vi "Untitled 2.vi"() -> ()   [LabVIEW 2012, in "filenames.lvlib"]
uses:
  filenames.lvlib
panel:
  in  "stop":bool
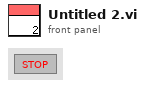
[diagram p1: front panel]
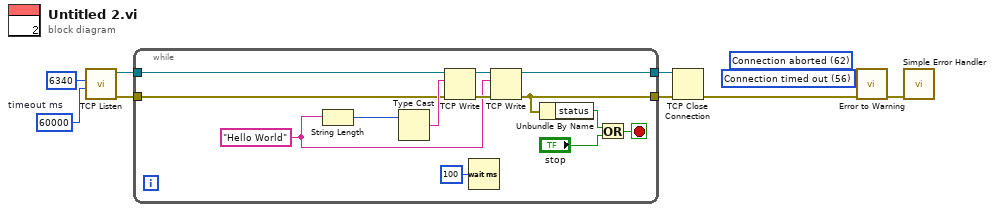
[diagram p0: block diagram]
diagram:
  w2 = 60000  # timeout ms
  w7 = 56 items=["No Error", "Argument Error", "Memory Full", "Out of Zone", "End of File", "File Already Open", "Generic File IO Error", "File Not Found", "File Permission Error", "Disk Full", "Duplicate Path", "Too Many Files Open", "Not Enabled", "Resource File Not Found", "Cannot Add Resource", "Resource Not Found", "Image Not Found", "Image Memory Error", "Pen Does Not Exist", "Config Bad Type", "Config Token Not Found", "Config Parse Error", "Config Memory Error", "Bad External Code Format", "Bad External Code Offset", "External Code Not Present", "Null Window", "Destroy Window Mixup", "Null Menu", "Print Aborted", "Bad Print Record", "Print Driver Error", "Windows Error During Print", "Memory Error During Print", "Print Dialog Error", "Generic Print Error", "Invalid Device Refnum", "Device Not Found", "Device Parameter Error", "Device Unit Error", "Can't Open Device", "Device Call Aborted", "Generic Error", "Cancelled By User", "Object ID Too Low", "Object ID Too High", "Object Not In Heap", "Unknown Heap", "Bad DefProc ID", "DefProc Not In Table", "Message Out Of Range", "Null Method", "Unknown Message", "Manager Call Not Supported", "Bad address", "Connection In progress", "Connection timed out", "Connection is already in progress", "Network attribute not supported", "Network error", "Address in use", "System out of memory", "Connection aborted", "Connection refused", "Connection is not connected", "Connection is already connected", "Connection closed", "Initialize error (interapplication manager)", "Bad occurrence", "Wait on unbound occurrence handler", "Occurrence queue overflow", "Bad path", "Semaphore not signaled", "Unrecognized type (interapplication manager)"] ("2nd Error to Convert")
  w8 = 62 items=["No Error", "Argument Error", "Memory Full", "Out of Zone", "End of File", "File Already Open", "Generic File IO Error", "File Not Found", "File Permission Error", "Disk Full", "Duplicate Path", "Too Many Files Open", "Not Enabled", "Resource File Not Found", "Cannot Add Resource", "Resource Not Found", "Image Not Found", "Image Memory Error", "Pen Does Not Exist", "Config Bad Type", "Config Token Not Found", "Config Parse Error", "Config Memory Error", "Bad External Code Format", "Bad External Code Offset", "External Code Not Present", "Null Window", "Destroy Window Mixup", "Null Menu", "Print Aborted", "Bad Print Record", "Print Driver Error", "Windows Error During Print", "Memory Error During Print", "Print Dialog Error", "Generic Print Error", "Invalid Device Refnum", "Device Not Found", "Device Parameter Error", "Device Unit Error", "Can't Open Device", "Device Call Aborted", "Generic Error", "Cancelled By User", "Object ID Too Low", "Object ID Too High", "Object Not In Heap", "Unknown Heap", "Bad DefProc ID", "DefProc Not In Table", "Message Out Of Range", "Null Method", "Unknown Message", "Manager Call Not Supported", "Bad address", "Connection In progress", "Connection timed out", "Connection is already in progress", "Network attribute not supported", "Network error", "Address in use", "System out of memory", "Connection aborted", "Connection refused", "Connection is not connected", "Connection is already connected", "Connection closed", "Initialize error (interapplication manager)", "Bad occurrence", "Wait on unbound occurrence handler", "Occurrence queue overflow", "Bad path", "Semaphore not signaled", "Unrecognized type (interapplication manager)"] ("1st Error to Convert")
  n1 = call <vilib>:"TCP Listen.vi"("timeout ms (wait forever: -1)"=w2, "port"=u16 6340) -> ("error out"=w3:errorcluster, "connection ID"=w5:refnum<k5>)  [unwired: 5 in, 3 out]
  n2 = while {
    tunnel: [w16] -> w4
    tunnel: [w23] -> w6
    tunnel: w5 -> [w22]
    tunnel: w3 -> [w13]
    stop <- w15 stop-if-true
    w11 = "Hello World" ("data in")
    n3 = String Length(string=w11) -> (length=w19:i32)
    n4 = Type Cast(x=w19) -> (*(type *) &x=w18:string)  [unwired: 1 in]
    n5 = TCP Write(connection ID=w22, data in=w18, error in (no error)=w13) -> (connection ID out=w21:refnum<k5>, error out=w20:errorcluster)  [unwired: 1 in, 1 out]
    n6 = Wait (ms)(milliseconds to wait=u32 100) -> ()  [unwired: 1 out]
    n7 = TCP Write(connection ID=w21, data in=w11, error in (no error)=w20) -> (connection ID out=w23:refnum<k5>, error out=w16:errorcluster)  [unwired: 1 in, 1 out]
    n8 = Unbundle By Name(w16) -> ("status"=w14:bool)
    n9 = Or(x=w14, y="stop") -> (x .or. y?=w15:bool)
  }
  n10 = TCP Close Connection(connection ID=w6, error in (no error)=w4) -> (error out=w10:errorcluster)  [unwired: 1 in, 1 out]
  n11 = call <vilib>:"Error to Warning.vi"("1st Error to Convert"=w8, "2nd Error to Convert"=w7, "error in"=w10) -> ("warning out"=w9:errorcluster)  [unwired: 12 in]
  n12 = call <vilib>:"Simple Error Handler.vi"("error in (no error)"=w9) -> ()  [unwired: 4 in, 5 out]
